vi "Terminal-Alert-ErrorTrigger.vi"(10 "报警信息":T1={"报警级别"="E0", "报警系统"="", "报警详情"="", "备注"=""}, 11 "error in (no error)":errorcluster caption="是否错误？") -> ()   [LabVIEW 2014]
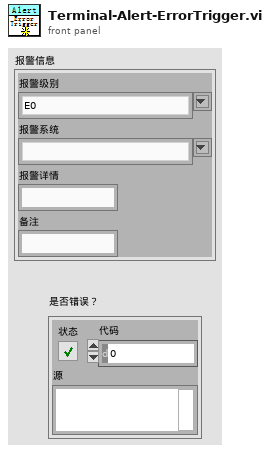
[diagram p1: front panel]
types:
  T1 = cluster{"报警级别":string, "报警系统":string, "报警详情":string, "备注":string}
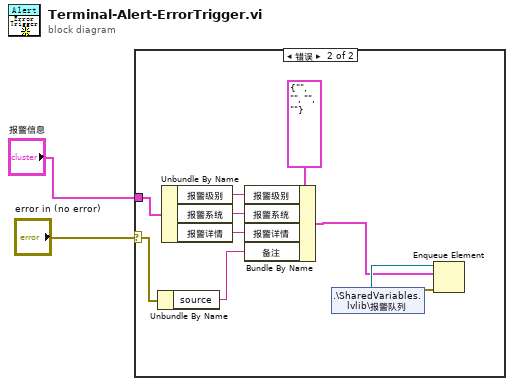
[diagram p0: block diagram]
diagram:
  n1 = case shown="错误" "error in (no error)" {
    selector: "error in (no error)" -> [_ w5]
    tunnel: "报警信息" -> [_ w9]
    frame No Error {
    }
    frame Error {
      n2 = Unbundle By Name(w5) -> ("source"=w4:string)
      n3 = Unbundle By Name(w9) -> ("报警级别"=w8:string, "报警系统"=w7:string, "报警详情"=w6:string)
      n4 = Bundle By Name(cluster=T1 {"报警级别"="", "报警系统"="", "报警详情"="", "备注"=""} ("报警信息"), "报警级别"=w8, "报警系统"=w7, "报警详情"=w6, "备注"=w4) -> (w3:T1)
      n5 = shared-variable ".\\SharedVariables.lvlib\\报警队列"() -> (w12:refnum<queue>, error out=w11:errorcluster)  [unwired: 1 in]
      n6 = Enqueue Element(queue=w12, element=w3, error in (no error)=w11) -> ()  [unwired: 1 in, 3 out]
    }
  }
